vi "Align to Base Buffer.vi"(8 "error in (no error)":errorcluster, 10 "base Buffer":refnum<class "Buffer.lvclass">, 11 "Buffer in":refnum<class "Buffer.lvclass">) -> (0 "error out":errorcluster, 3 "Buffer out":refnum<class "Buffer.lvclass">)   [LabVIEW 2017, in "DSF Core.lvlib" / "Buffer.lvclass"]
doc: "Offsets <b>Buffer</b> using its configured buffer offset to an address that is offset from the provided <b>base Buffer</b>.\n\nThe offset <b>Buffer</b> must be within the bounds of <b>base Buffer</b>."
uses:
  Buffer.lvclass
  C:/Program Files (x86)/National Instruments/LabVIEW 2017/vi.lib/NI/Memory Manager/Classes/Pointer/Pointer.lvclass
  <vilib>/NI/Memory Manager/Classes/Pointer/Pointer.lvclass/Pointer.ctl
  Buffer.lvclass/Buffer.ctl
  <vilib>/NI/Memory Manager/Classes/Pointer/Set Size.vi
  <vilib>/NI/Memory Manager/Classes/Pointer/Set Address.vi
  <vilib>/NI/Memory Manager/Classes/Pointer/Check Null Pointer.vi
  <vilib>/NI/Memory Manager/Classes/Pointer/Set Internal.vi
  <vilib>/NI/Memory Manager/Classes/Pointer/Errors.vi
  <vilib>/NI/Memory Manager/Classes/Pointer/Null Pointer.vi
  <vilib>/NI/Memory Manager/Classes/Pointer/Create Error.vi
  <vilib>/NI/Memory Manager/VIs/New Error Cluster Constant.vi
  <vilib>/NI/Memory Manager/VIs/New Error Cluster Constant (512B).vi
  <vilib>/NI/Memory Manager/VIs/Error Cluster.Set Status.vi
  <vilib>/NI/Memory Manager/VIs/Error Cluster.Set Code.vi
  <vilib>/NI/Memory Manager/VIs/Error Cluster.Set VI Source.vi
  <vilib>/NI/Memory Manager/Constants/Constants.vi
  <vilib>/NI/Memory Manager/Constants/Library Name.vi
  <vilib>/NI/Memory Manager/Classes/Pointer/Pointer Error Info.vi
  <vilib>/NI/Memory Manager/VIs/Source.Write.String.vi
  <vilib>/NI/Memory Manager/Constants/Pointer Class Name.vi
  <vilib>/NI/Memory Manager/Classes/Pointer/Pointer.lvclass
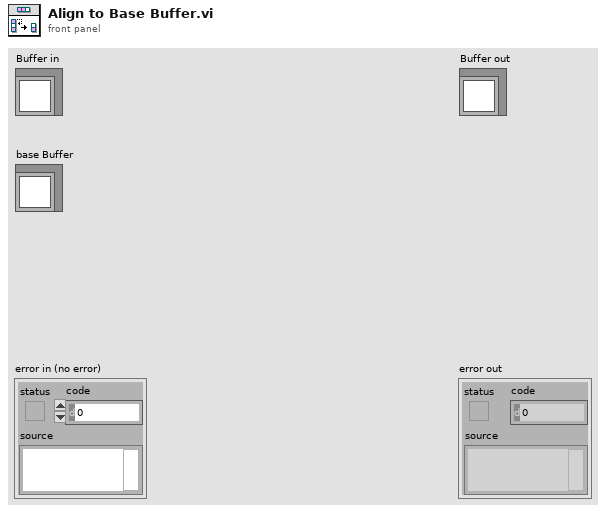
[diagram p1: front panel]
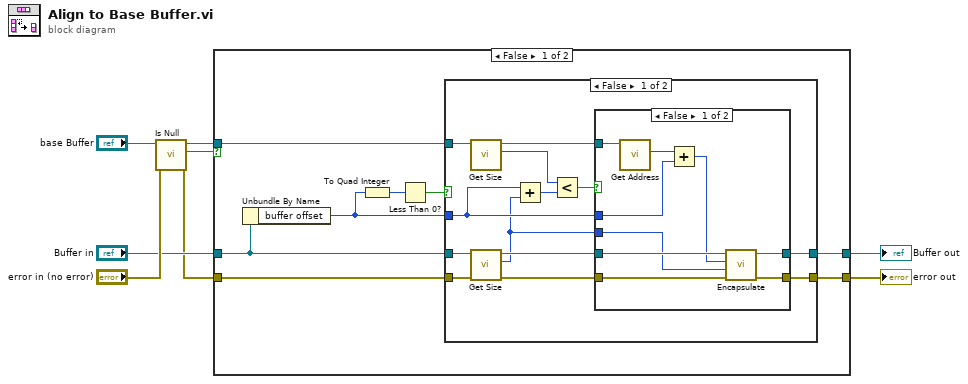
[diagram p0: block diagram]
diagram:
  n1 = call <vilib>:"Is Null.vi"("error in (no error)"="error in (no error)", "Pointer in"="base Buffer") -> ("error out"=w2:errorcluster, "null?"=w1:bool, "Pointer out"=w3:refnum<class "Buffer.lvclass">)  [unwired: 7 in]
  n2 = case shown="False" w1 {
    tunnel: [w16 w43] -> w8
    tunnel: [w15 w42] -> w7
    tunnel: w3 -> [w11 _]
    tunnel: "Buffer in" -> [w9 w43]
    tunnel: w2 -> [w10 w42]
    frame False {
      n3 = Unbundle By Name(w9) -> ("buffer offset"=w14:u64)
      n4 = To Quad Integer(1:w14) -> (0:w13:i64)
      n5 = Less Than 0?(x=w13) -> (x < 0?=w12:bool)
      n6 = case shown="False" w12 {
        tunnel: [w28 w40] -> w16
        tunnel: [w27 w41] -> w15
        tunnel: w10 -> [w26 w41]
        tunnel: w9 -> [w19 w40]
        tunnel: w14 -> [w25 _]
        tunnel: w11 -> [w22 _]
        frame False {
          n7 = call <vilib>:"Get Size.vi"("Pointer in"=w22) -> ("size"=w20:u64, "Pointer out"=w21:refnum<class "Buffer.lvclass">)  [unwired: 9 in]
          n8 = call <vilib>:"Get Size.vi"("Pointer in"=w19) -> ("size"=w17:u64, "Pointer out"=w18:refnum<class "Buffer.lvclass">)  [unwired: 9 in]
          n9 = Add(x=w25, y=w17) -> (x+y=w24:u64)
          n10 = Less?(x=w20, y=w24) -> (x < y?=w23:bool)
          n11 = case shown="False" w23 {
            tunnel: [w37 w38] -> w28
            tunnel: [w36 w39] -> w27
            tunnel: w26 -> [w35 w39]
            tunnel: w18 -> [w34 w38]
            tunnel: w17 -> [w33 _]
            tunnel: w25 -> [w31 _]
            tunnel: w21 -> [w30 _]
            frame False {
              n12 = call <vilib>:"Get Address.vi"("Pointer in"=w30) -> ("address"=w29:u64)  [unwired: 9 in, 1 out]
              n13 = Add(x=w29, y=w31) -> (x+y=w32:u64)
              n14 = call <vilib>:"Encapsulate.vi"("error in (no error)"=w35, "size"=w33, "address"=w32, "Pointer in"=w34) -> ("error out"=w36:errorcluster, "Pointer out"=w37:refnum<class "Buffer.lvclass">)  [unwired: 6 in]
            }
            frame True {
              # "offset would be out of bounds of base buffer."
            }
          }
        }
        frame True {
          # "invalid offset"
        }
      }
    }
    frame True {
    }
  }
  "error out" <- w7
  "Buffer out" <- w8
